vi "Reconstruct_Special_Case_101-Empty-2.vi"(4 "[IN] Index of \nBest Subtrack":i32, 6 "[IN] Subtracks":T1(array[cluster]), 8 "error IN":errorcluster, 9 "[IN] Indicies of sub\ntracks for transforma\ntion (resolving)":i32[](array[numeric]), 10 "[IN] Clusters for Re\nconstructed Tracks":T3, 11 "[IN] Still connected\ntracks in group":T2) -> (0 "error OUT":errorcluster, 2 "[OUT] Clusters for Re\nconstructed Tracks":T3)   [LabVIEW 2013]
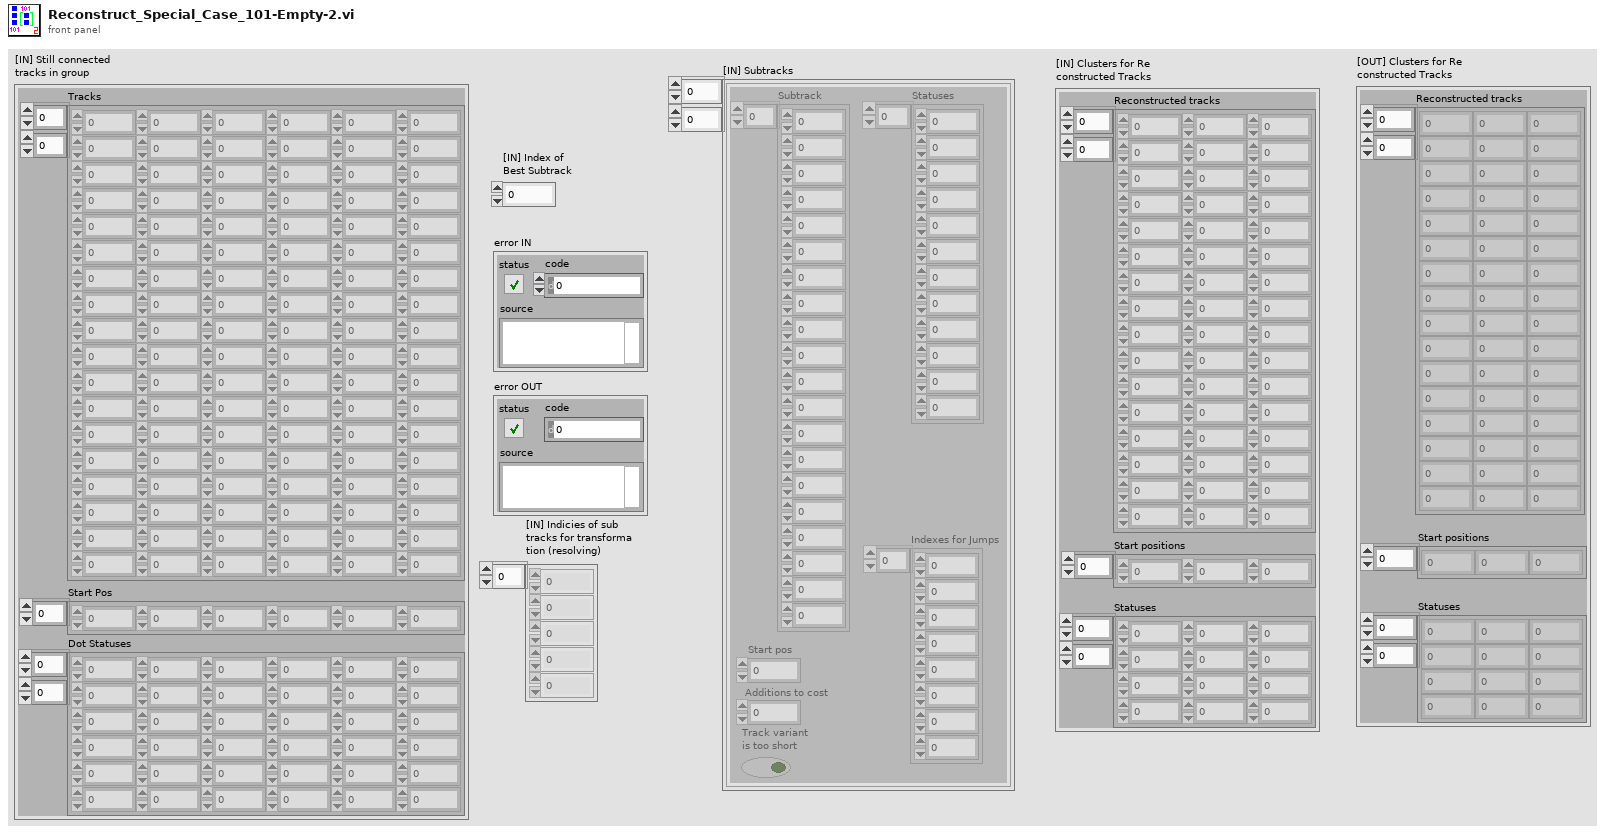
[diagram p1: front panel]
types:
  T1 = cluster{"Subtrack":dbl[], "Statuses":i16[], "Start pos":i32, "Additions to cost":i32, "Track variant \nis too short":bool, "Indexes for Jumps":i32[]}[][]
  T2 = cluster{"Tracks":dbl[][], "Start Pos":i32[], "Dot Statuses":i16[][]}
  T3 = cluster{"Reconstructed tracks":dbl[][], "Start positions":i32[], "Statuses":i16[][]}
  T4 = cluster{"Subtrack":dbl[], "Statuses":i16[], "Start pos":i32, "Additions to cost":i32, "Track variant \nis too short":bool, "Indexes for Jumps":i32[]}
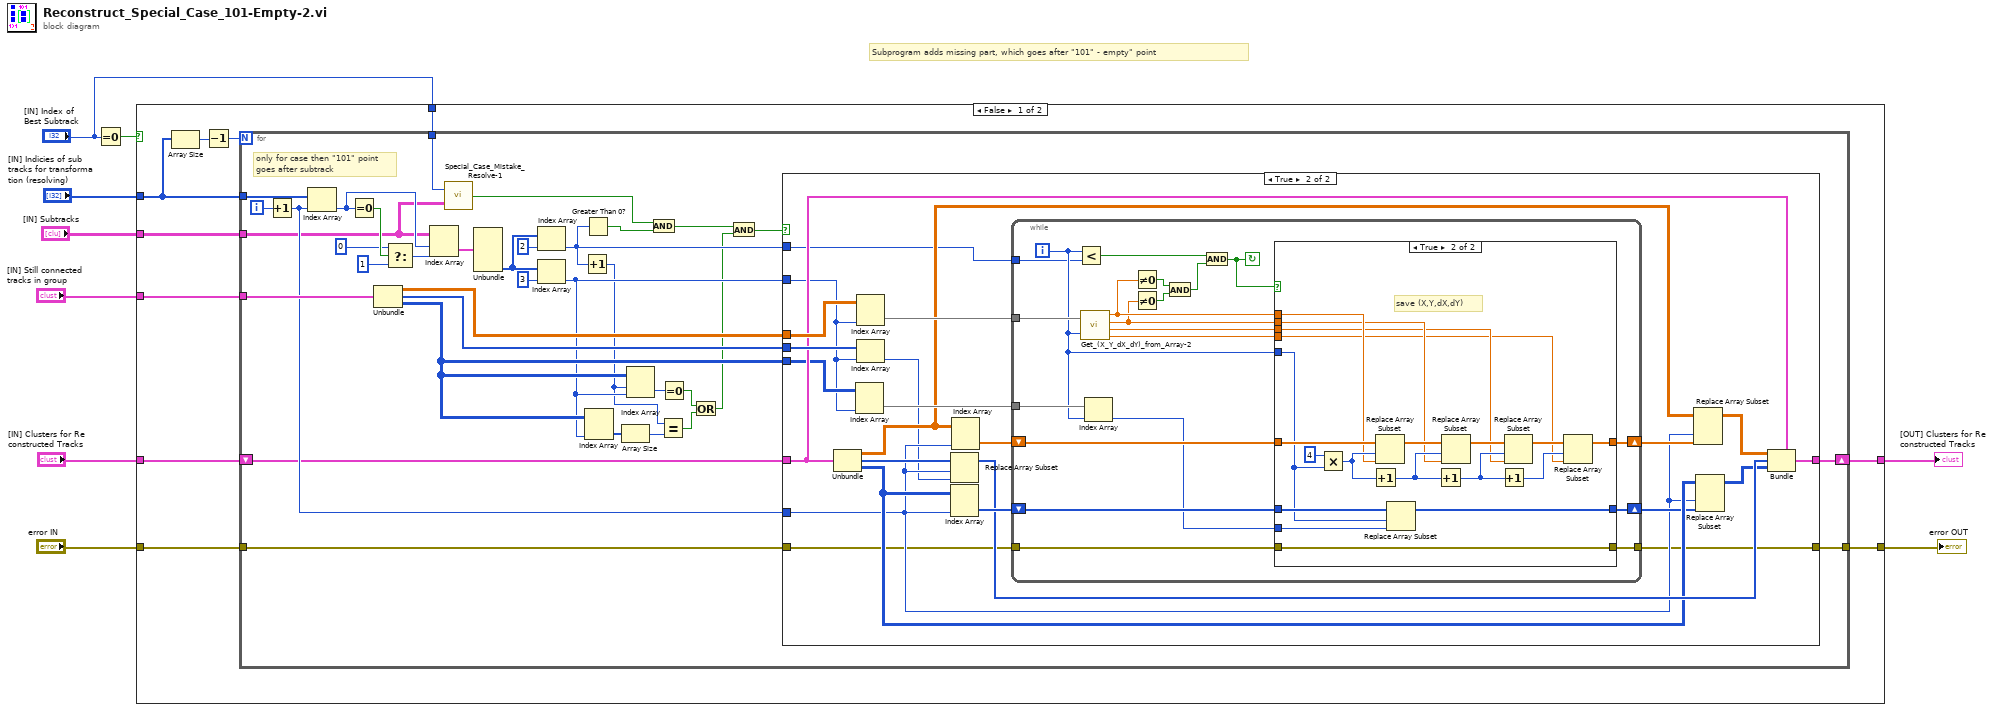
[diagram p0: block diagram]
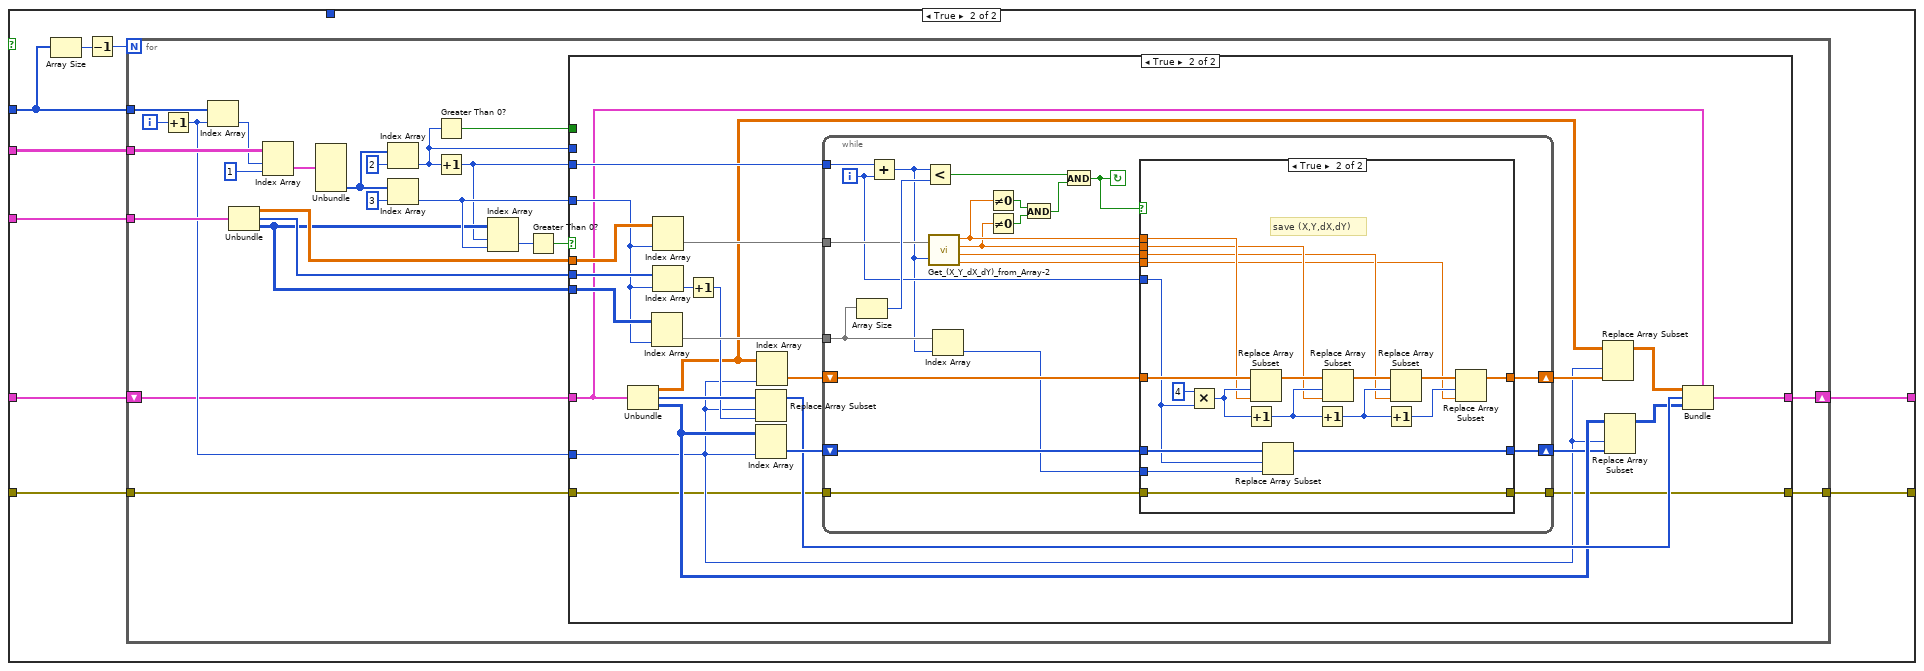
[diagram p4: hidden frame]
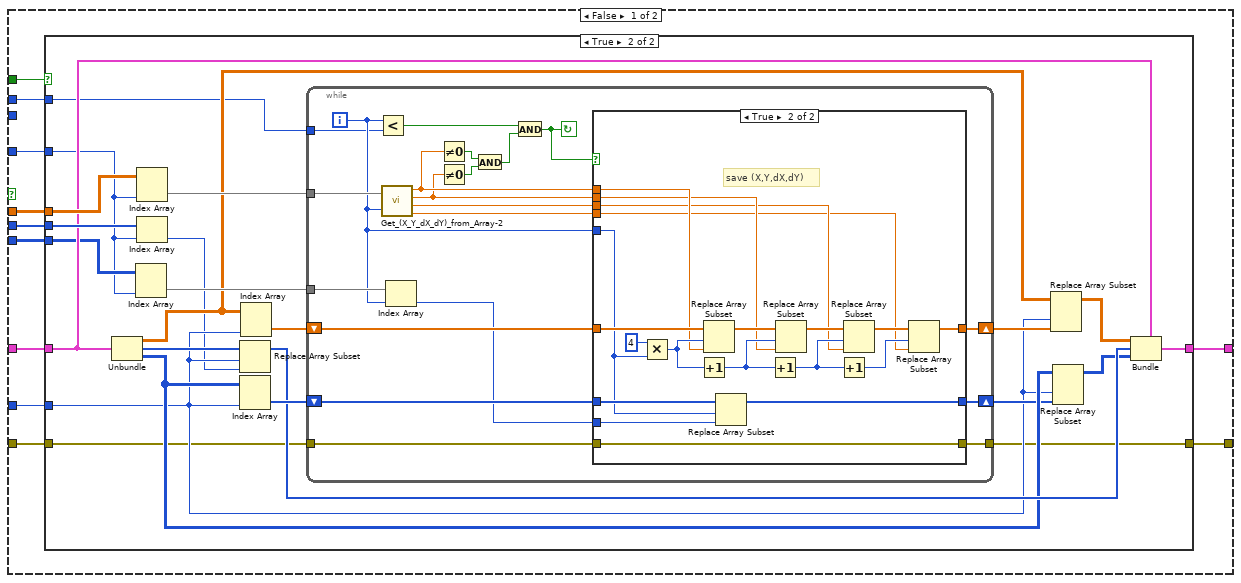
[diagram p5: hidden frame]
diagram:
  # "Subprogram adds missing part, which goes after \"101\" - empty\" point"
  n1 = Equal To 0?(x="[IN] Index of \nBest Subtrack") -> (x = 0?=w9:bool)
  n2 = case shown="False" w9 {
    tunnel: "[IN] Indicies of sub\ntracks for transforma\ntion (resolving)" -> [w13 w128]
    tunnel: "[IN] Subtracks" -> [w14 w127]
    tunnel: "[IN] Still connected\ntracks in group" -> [w15 w126]
    tunnel: "[IN] Clusters for Re\nconstructed Tracks" -> [w17 w125]
    tunnel: "error IN" -> [w16 w124]
    tunnel: [w12 w123] -> w3
    tunnel: [w11 w122] -> w2
    tunnel: "[IN] Index of \nBest Subtrack" -> [w10 _]
    frame False {
      n3 = Array Size(array=w13) -> (size(s)=w19:i32)
      n4 = Decrement(x=w19) -> (x-1=w18:i32)
      n5 = for {
        N: w18 -> [_]
        tunnel: w13 -> [w54]
        tunnel: w14 -> [w22]
        tunnel: w15 -> [w49]
        shift-right: [w46] -> w12
        shift-left: w17 -> [w47]
        tunnel: w16 -> [w43]
        tunnel: [w42] -> w11
        tunnel: w10 -> [w23]
        i -> [w53]
        # "only for case then \"101\" point\ngoes after subtrack"
        n6 = Increment(x=w53) -> (x+1=w48:i32)
        n7 = Index Array(array=w54, index=w48) -> (element=w26:i32)
        n8 = Equal To 0?(x=w26) -> (x = 0?=w30:bool)
        n9 = Unbundle(w49) -> ("Tracks"=w45:dbl[][], "Start Pos"=w44:i32[], "Dot Statuses"=w38:i16[][])
        n10 = Select(t=0 ("disabled index (col)"), s=w30, f=1 ("disabled index (col)")) -> (s? t:f=w27:i32)
        n11 = Index Array(array=w22, index (row)=w26, index (col)=w27) -> (element=w52:T4)
        n12 = call "Special_Case_Mistake_Resolve-1.vi"("[IN] Subtracks"=w22, "[IN] Index of \nBest Subtrack"=w23) -> ("[OUT] FALSE For Pre\nventing double save"=w21:bool)
        n13 = Unbundle(w52) -> ("Indexes for Jumps"=w41:i32[])  [unwired: 5 out]
        n14 = Index Array(array=w41, index=2) -> (element=w40:i32)
        n15 = Index Array(array=w41, index=3) -> (element=w37:i32)
        n16 = Increment(x=w40) -> (x+1=w34:i32)
        n17 = Greater Than 0?(x=w40) -> (x > 0?=w25:bool)
        n18 = Index Array(array=w38, index (col)=w37) -> (element=w36:i16[])  [unwired: 1 in]
        n19 = Array Size(array=w36) -> (size(s)=w35:i32)
        n20 = Index Array(array=w38, index (row)=w34, index (col)=w37) -> (element=w39:i16)
        n21 = And(x=w21, y=w25) -> (x .and. y?=w24:bool)
        n22 = Equal?(x=w34, y=w35) -> (x = y?=w33:bool)
        n23 = Equal To 0?(x=w39) -> (x = 0?=w32:bool)
        n24 = Or(x=w32, y=w33) -> (x .or. y?=w31:bool)
        n25 = And(x=w24, y=w31) -> (x .and. y?=w20:bool)
        n26 = case shown="True" w20 {
          tunnel: w45 -> [_ w67]
          tunnel: w44 -> [_ w66]
          tunnel: w47 -> [w56 w65]
          tunnel: w48 -> [_ w64]
          tunnel: w43 -> [w55 w63]
          tunnel: w38 -> [_ w62]
          tunnel: w37 -> [_ w61]
          tunnel: w40 -> [_ w60]
          tunnel: [w56 w58] -> w46
          tunnel: [w55 w57] -> w42
          frame False {
          }
          frame True {
            n27 = Unbundle(w65) -> ("Reconstructed tracks"=w73:dbl[][], "Start positions"=w79:i32[], "Statuses"=w70:i16[][])
            n28 = Index Array(array=w62, index (col)=w61) -> (element=w78:i16[])  [unwired: 1 in]
            n29 = Index Array(array=w67, index (col)=w61) -> (element=w77:dbl[])  [unwired: 1 in]
            n30 = Index Array(array=w66, index=w61) -> (element=w59:i32)
            n31 = Replace Array Subset(array=w79, new element=w59, index=w64) -> (w71:i32[])
            n32 = Index Array(array=w70, index (col)=w64) -> (element=w75:i16[])  [unwired: 1 in]
            n33 = Index Array(array=w73, index (col)=w64) -> (element=w76:dbl[])  [unwired: 1 in]
            n34 = while {
              tunnel: w78 -> [w86]
              tunnel: w77 -> [w99]
              shift-right: [w87] -> w74
              shift-left: w76 -> [w92]
              shift-right: [w84] -> w69
              shift-left: w75 -> [w93]
              tunnel: w63 -> [w83]
              tunnel: [w82] -> w57
              tunnel: w60 -> [w80]
              i -> [w81]
              stop <- w94 continue-if-true
              n35 = Less?(x=w81, y=w80) -> (x < y?=w96:bool)
              n36 = call "Get_(X_Y_dX_dY)_from_Array-2.vi"("(X,Y,dX,dY)"=w99, "Index of Displacement"=w81) -> ("X"=w91:dbl, "Y"=w90:dbl, "dX"=w89:dbl, "dY"=w88:dbl)
              n37 = Index Array(array=w86, index=w81) -> (element=w85:i16)
              n38 = Not Equal To 0?(x=w91) -> (x != 0?=w98:bool)
              n39 = Not Equal To 0?(x=w90) -> (x != 0?=w97:bool)
              n40 = And(x=w98, y=w97) -> (x .and. y?=w95:bool)
              n41 = And(x=w96, y=w95) -> (x .and. y?=w94:bool)
              n42 = case shown="True" w94 {
                tunnel: w93 -> [w101 w107]
                tunnel: w92 -> [w102 w117]
                tunnel: w81 -> [_ w106]
                tunnel: w91 -> [_ w112]
                tunnel: w90 -> [_ w111]
                tunnel: w89 -> [_ w110]
                tunnel: w88 -> [_ w109]
                tunnel: [w102 w108] -> w87
                tunnel: w85 -> [_ w105]
                tunnel: [w101 w104] -> w84
                tunnel: w83 -> [w100 w103]
                tunnel: [w100 w103] -> w82
                frame False {
                }
                frame True {
                  # "save (X,Y,dX,dY)"
                  n43 = Multiply(x=4, y=w106) -> (x*y=w116:i32)
                  n44 = Increment(x=w116) -> (x+1=w115:i32)
                  n45 = Replace Array Subset(array=w117, new element=w112, index=w116) -> (w120:dbl[])
                  n46 = Replace Array Subset(array=w107, new element=w105, index=w106) -> (w104:i16[])
                  n47 = Increment(x=w115) -> (x+1=w114:i32)
                  n48 = Replace Array Subset(array=w120, new element=w111, index=w115) -> (w119:dbl[])
                  n49 = Increment(x=w114) -> (x+1=w113:i32)
                  n50 = Replace Array Subset(array=w119, new element=w110, index=w114) -> (w118:dbl[])
                  n51 = Replace Array Subset(array=w118, new element=w109, index=w113) -> (w108:dbl[])
                }
              }
            }
            n52 = Replace Array Subset(array=w73, new element=w74, index (col)=w64) -> (w72:dbl[][])  [unwired: 1 in]
            n53 = Replace Array Subset(array=w70, new element=w69, index (col)=w64) -> (w68:i16[][])  [unwired: 1 in]
            n54 = Bundle(cluster=w65, "Reconstructed tracks"=w72, "Start positions"=w71, "Statuses"=w68) -> (w58:T3)
          }
        }
      }
    }
    frame True {
      n55 = Array Size(array=w128) -> (size(s)=w130:i32)
      n56 = Decrement(x=w130) -> (x-1=w129:i32)
      n57 = for {
        N: w129 -> [_]
        tunnel: w128 -> [w154]
        tunnel: w127 -> [w152]
        tunnel: w126 -> [w146]
        shift-right: [w141] -> w123
        shift-left: w125 -> [w142]
        tunnel: w124 -> [w136]
        tunnel: [w135] -> w122
        i -> [w153]
        n58 = Increment(x=w153) -> (x+1=w144:i32)
        n59 = Index Array(array=w154, index=w144) -> (element=w150:i32)
        n60 = Unbundle(w146) -> ("Tracks"=w140:dbl[][], "Start Pos"=w139:i32[], "Dot Statuses"=w138:i16[][])
        n61 = Index Array(array=w152, index (row)=w150, index (col)=1 ("disabled index (col)")) -> (element=w149:T4)
        n62 = Unbundle(w149) -> ("Indexes for Jumps"=w134:i32[])  [unwired: 5 out]
        n63 = Index Array(array=w134, index=2) -> (element=w131:i32)
        n64 = Index Array(array=w134, index=3) -> (element=w143:i32)
        n65 = Greater Than 0?(x=w131) -> (x > 0?=w132:bool)
        n66 = Increment(x=w131) -> (x+1=w137:i32)
        n67 = Index Array(array=w138, index (row)=w137, index (col)=w143) -> (element=w133:i16)
        n68 = Greater Than 0?(x=w133) -> (x > 0?=w145:bool)
        n69 = case shown="True" w145 {
          tunnel: w144 -> [w162 w236]
          tunnel: w143 -> [w159 w251]
          tunnel: w142 -> [w163 w244]
          tunnel: [w156 w240] -> w141
          tunnel: w140 -> [w165 w253]
          tunnel: w139 -> [w164 w255]
          tunnel: w138 -> [w160 w252]
          tunnel: w137 -> [_ w248]
          tunnel: w136 -> [w161 w234]
          tunnel: [w155 w233] -> w135
          tunnel: w132 -> [w158 _]
          tunnel: w131 -> [w157 _]
          frame False {
            n70 = case shown="True" w158 {
              tunnel: w165 -> [_ w178]
              tunnel: w164 -> [_ w177]
              tunnel: w163 -> [w167 w176]
              tunnel: w162 -> [_ w175]
              tunnel: w161 -> [w166 w174]
              tunnel: w160 -> [_ w173]
              tunnel: w159 -> [_ w172]
              tunnel: w157 -> [_ w171]
              tunnel: [w167 w169] -> w156
              tunnel: [w166 w168] -> w155
              frame False {
              }
              frame True {
                n71 = Unbundle(w176) -> ("Reconstructed tracks"=w184:dbl[][], "Start positions"=w190:i32[], "Statuses"=w181:i16[][])
                n72 = Index Array(array=w173, index (col)=w172) -> (element=w189:i16[])  [unwired: 1 in]
                n73 = Index Array(array=w178, index (col)=w172) -> (element=w188:dbl[])  [unwired: 1 in]
                n74 = Index Array(array=w177, index=w172) -> (element=w170:i32)
                n75 = Replace Array Subset(array=w190, new element=w170, index=w175) -> (w182:i32[])
                n76 = Index Array(array=w181, index (col)=w175) -> (element=w186:i16[])  [unwired: 1 in]
                n77 = Index Array(array=w184, index (col)=w175) -> (element=w187:dbl[])  [unwired: 1 in]
                n78 = while {
                  tunnel: w189 -> [w197]
                  tunnel: w188 -> [w210]
                  shift-right: [w198] -> w185
                  shift-left: w187 -> [w203]
                  shift-right: [w195] -> w180
                  shift-left: w186 -> [w204]
                  tunnel: w174 -> [w194]
                  tunnel: [w193] -> w168
                  tunnel: w171 -> [w191]
                  i -> [w192]
                  stop <- w205 continue-if-true
                  n79 = Less?(x=w192, y=w191) -> (x < y?=w207:bool)
                  n80 = call "Get_(X_Y_dX_dY)_from_Array-2.vi"("(X,Y,dX,dY)"=w210, "Index of Displacement"=w192) -> ("X"=w202:dbl, "Y"=w201:dbl, "dX"=w200:dbl, "dY"=w199:dbl)
                  n81 = Index Array(array=w197, index=w192) -> (element=w196:i16)
                  n82 = Not Equal To 0?(x=w202) -> (x != 0?=w209:bool)
                  n83 = Not Equal To 0?(x=w201) -> (x != 0?=w208:bool)
                  n84 = And(x=w209, y=w208) -> (x .and. y?=w206:bool)
                  n85 = And(x=w207, y=w206) -> (x .and. y?=w205:bool)
                  n86 = case shown="True" w205 {
                    tunnel: w204 -> [w212 w218]
                    tunnel: w203 -> [w213 w228]
                    tunnel: w192 -> [_ w217]
                    tunnel: w202 -> [_ w223]
                    tunnel: w201 -> [_ w222]
                    tunnel: w200 -> [_ w221]
                    tunnel: w199 -> [_ w220]
                    tunnel: [w213 w219] -> w198
                    tunnel: w196 -> [_ w216]
                    tunnel: [w212 w215] -> w195
                    tunnel: w194 -> [w211 w214]
                    tunnel: [w211 w214] -> w193
                    frame False {
                    }
                    frame True {
                      # "save (X,Y,dX,dY)"
                      n87 = Multiply(x=4, y=w217) -> (x*y=w227:i32)
                      n88 = Increment(x=w227) -> (x+1=w226:i32)
                      n89 = Replace Array Subset(array=w228, new element=w223, index=w227) -> (w231:dbl[])
                      n90 = Replace Array Subset(array=w218, new element=w216, index=w217) -> (w215:i16[])
                      n91 = Increment(x=w226) -> (x+1=w225:i32)
                      n92 = Replace Array Subset(array=w231, new element=w222, index=w226) -> (w230:dbl[])
                      n93 = Increment(x=w225) -> (x+1=w224:i32)
                      n94 = Replace Array Subset(array=w230, new element=w221, index=w225) -> (w229:dbl[])
                      n95 = Replace Array Subset(array=w229, new element=w220, index=w224) -> (w219:dbl[])
                    }
                  }
                }
                n96 = Replace Array Subset(array=w184, new element=w185, index (col)=w175) -> (w183:dbl[][])  [unwired: 1 in]
                n97 = Replace Array Subset(array=w181, new element=w180, index (col)=w175) -> (w179:i16[][])  [unwired: 1 in]
                n98 = Bundle(cluster=w176, "Reconstructed tracks"=w183, "Start positions"=w182, "Statuses"=w179) -> (w169:T3)
              }
            }
          }
          frame True {
            n99 = Unbundle(w244) -> ("Reconstructed tracks"=w242:dbl[][], "Start positions"=w256:i32[], "Statuses"=w238:i16[][])
            n100 = Index Array(array=w252, index (col)=w251) -> (element=w250:i16[])  [unwired: 1 in]
            n101 = Index Array(array=w253, index (col)=w251) -> (element=w249:dbl[])  [unwired: 1 in]
            n102 = Index Array(array=w255, index=w251) -> (element=w254:i32)
            n103 = Increment(x=w254) -> (x+1=w247:i32)
            n104 = Replace Array Subset(array=w256, new element=w247, index=w236) -> (w239:i32[])
            n105 = Index Array(array=w238, index (col)=w236) -> (element=w245:i16[])  [unwired: 1 in]
            n106 = Index Array(array=w242, index (col)=w236) -> (element=w246:dbl[])  [unwired: 1 in]
            n107 = while {
              tunnel: w250 -> [w262]
              tunnel: w249 -> [w276]
              tunnel: w248 -> [w278]
              shift-right: [w263] -> w243
              shift-left: w246 -> [w269]
              shift-right: [w259] -> w237
              shift-left: w245 -> [w270]
              tunnel: w234 -> [w258]
              tunnel: [w257] -> w233
              i -> [w268]
              stop <- w271 continue-if-true
              n108 = Array Size(array=w262) -> (size(s)=w277:i32)
              n109 = Add(x=w278, y=w268) -> (x+y=w261:i32)
              n110 = Less?(x=w261, y=w277) -> (x < y?=w273:bool)
              n111 = call "Get_(X_Y_dX_dY)_from_Array-2.vi"("(X,Y,dX,dY)"=w276, "Index of Displacement"=w261) -> ("X"=w267:dbl, "Y"=w266:dbl, "dX"=w265:dbl, "dY"=w264:dbl)
              n112 = Index Array(array=w262, index=w261) -> (element=w260:i16)
              n113 = Not Equal To 0?(x=w267) -> (x != 0?=w275:bool)
              n114 = Not Equal To 0?(x=w266) -> (x != 0?=w274:bool)
              n115 = And(x=w275, y=w274) -> (x .and. y?=w272:bool)
              n116 = And(x=w273, y=w272) -> (x .and. y?=w271:bool)
              n117 = case shown="True" w271 {
                tunnel: w270 -> [w280 w286]
                tunnel: w269 -> [w281 w296]
                tunnel: w268 -> [_ w285]
                tunnel: w267 -> [_ w291]
                tunnel: w266 -> [_ w290]
                tunnel: w265 -> [_ w289]
                tunnel: w264 -> [_ w288]
                tunnel: [w281 w287] -> w263
                tunnel: w260 -> [_ w284]
                tunnel: [w280 w283] -> w259
                tunnel: w258 -> [w279 w282]
                tunnel: [w279 w282] -> w257
                frame False {
                }
                frame True {
                  # "save (X,Y,dX,dY)"
                  n118 = Multiply(x=4, y=w285) -> (x*y=w295:i32)
                  n119 = Increment(x=w295) -> (x+1=w294:i32)
                  n120 = Replace Array Subset(array=w296, new element=w291, index=w295) -> (w299:dbl[])
                  n121 = Replace Array Subset(array=w286, new element=w284, index=w285) -> (w283:i16[])
                  n122 = Increment(x=w294) -> (x+1=w293:i32)
                  n123 = Replace Array Subset(array=w299, new element=w290, index=w294) -> (w298:dbl[])
                  n124 = Increment(x=w293) -> (x+1=w292:i32)
                  n125 = Replace Array Subset(array=w298, new element=w289, index=w293) -> (w297:dbl[])
                  n126 = Replace Array Subset(array=w297, new element=w288, index=w292) -> (w287:dbl[])
                }
              }
            }
            n127 = Replace Array Subset(array=w242, new element=w243, index (col)=w236) -> (w241:dbl[][])  [unwired: 1 in]
            n128 = Replace Array Subset(array=w238, new element=w237, index (col)=w236) -> (w235:i16[][])  [unwired: 1 in]
            n129 = Bundle(cluster=w244, "Reconstructed tracks"=w241, "Start positions"=w239, "Statuses"=w235) -> (w240:T3)
          }
        }
      }
    }
  }
  "[OUT] Clusters for Re\nconstructed Tracks" <- w3
  "error OUT" <- w2
